vi "Sepios_DepthController_main-for separate Testing.vi"() -> ()   [LabVIEW 2013]
uses:
  <vilib>/myRIO/Instrument Drivers/Utilities/Utilities.lvlib
panel:
  in  "Excessive_Depth_Deviation_Trigger":dbl=0.4
  out "X_Actual [m]":dbl
  out "X_Desired":dbl
  in  "Calibrate Depth":bool
  out "P_ref [Pa]":dbl
  in  "Neutral Buoancy_x":dbl=0.2
  in  "Ti_Depth_Control":dbl=1e-05
  in  "kp_Depth_Control":dbl=0.3
  in  "Integrator enabled range Depth":dbl=0.1
  in  "kp_Motor":dbl=150.0 min=0.0 max=20.0 step=0.01
  in  "Ti_Motor":dbl=1.72e-05 min=0.0 step=0.0001
  in  "Integrator_enable_Range_Motor":dbl=0.03 min=0.0 step=0.01
  out "error out":errorcluster
  in  "STOP":bool
  in  "Tab Control":enum32{"Page 1"}(tab)
  in  "Max Depth":dbl=3.5 max=10.0 step=0.5
  out "Depth [m]":cluster{dbl, dbl, dbl}(slide)={0.0, -0.9890109890109892, 0.0} scale format="%#_3g"
  out "Motor Current[A]":dbl(knob) scale=0.0..3.0
  in  "Depth Desired [m]":dbl min=0.0 step=0.1
  # "Depth Conrol"
  # "SB: Position Control"
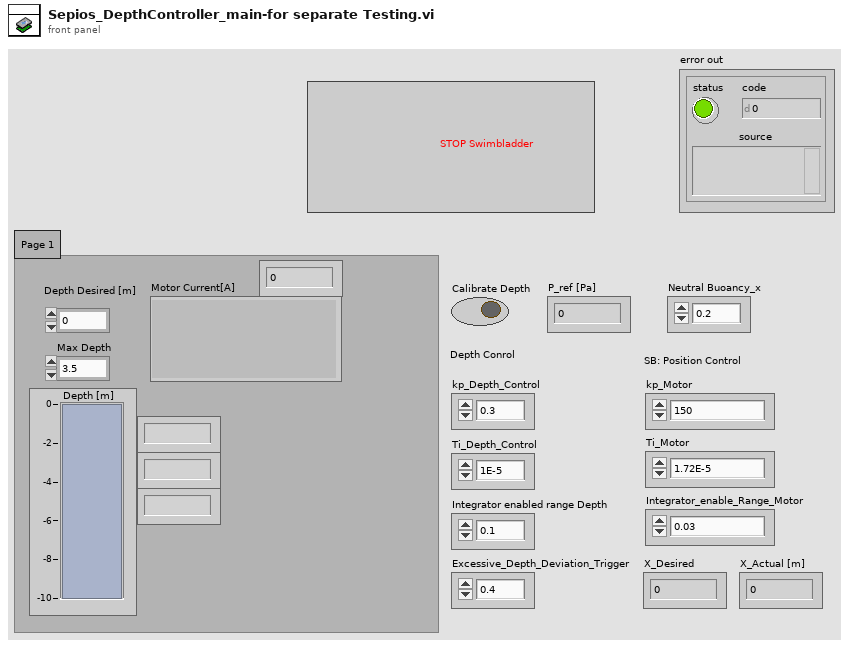
[diagram p1: front panel]
types:
  T1 = cluster{"Water Density":dbl, "SB_parameters":cluster{"x0":dbl, "U_full":dbl, "U_empty":dbl}}
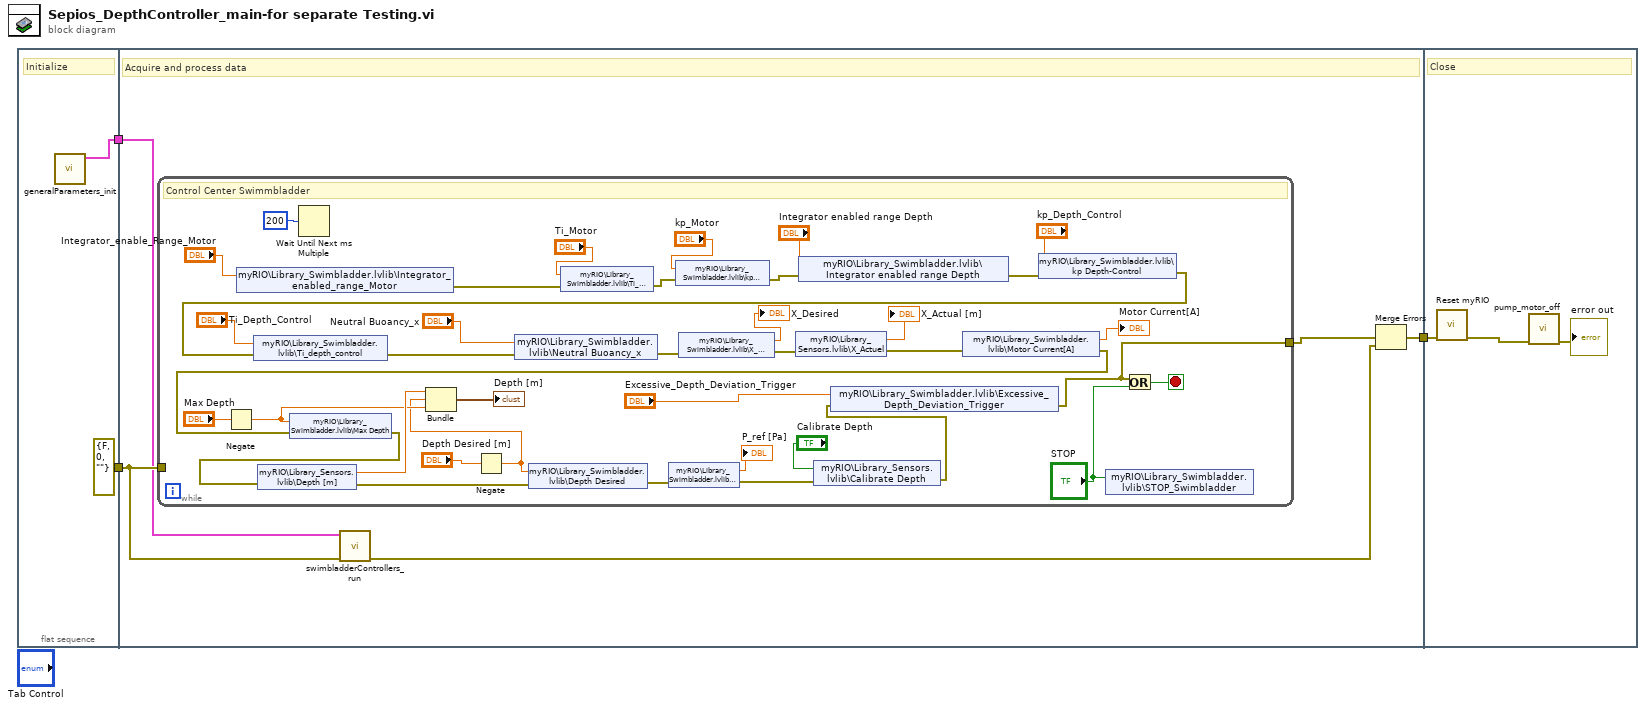
[diagram p0: block diagram]
diagram:
  n1 = flat-sequence {
    tunnel: [errorcluster {"status"=FALSE, "code"=0, "source"=""} ("error out")] -> w3
    tunnel: [w4] -> w2
    tunnel: w3 -> [w8]
    tunnel: w2 -> [w6]
    tunnel: [w10] -> w1
    tunnel: w1 -> [w51]
    frame #0 {
      # "Initialize"
      n2 = call "generalParameters_init.vi"() -> ("General Parameters"=w4:T1)  [unwired: 11 in]
    }
    frame #1 {
      # "Acquire and process data"
      n3 = while {
        tunnel: w8 -> [_]
        tunnel: [w12] -> w7
        stop <- w47 stop-if-true
        # "Control Center Swimmbladder"
        n4 = Negate(x="Max Depth") -> (-x=w15:dbl)
        n5 = shared-variable "myRIO\\Library_Swimbladder.lvlib\\Integrator_enabled_range_Motor"("Integrator_enable_Range_Motor") -> (error out=w41:errorcluster)  [unwired: 1 in]
        n6 = Wait Until Next ms Multiple(millisecond multiple=u32 200) -> ()  [unwired: 1 out]
        n7 = Negate(x="Depth Desired [m]") -> (-x=w14:dbl)
        n8 = shared-variable "myRIO\\Library_Swimbladder.lvlib\\Ti_Motor"("Ti_Motor", error in=w41) -> (error out=w40:errorcluster)
        n9 = shared-variable "myRIO\\Library_Swimbladder.lvlib\\kp Motor"("kp_Motor", error in=w40) -> (error out=w38:errorcluster)
        n10 = shared-variable "myRIO\\Library_Swimbladder.lvlib\\Integrator enabled range Depth"("Integrator enabled range Depth", error in=w38) -> (error out=w37:errorcluster)
        n11 = shared-variable "myRIO\\Library_Swimbladder.lvlib\\kp Depth-Control"("kp_Depth_Control", error in=w37) -> (error out=w35:errorcluster)
        n12 = shared-variable "myRIO\\Library_Swimbladder.lvlib\\Ti_depth_control"("Ti_Depth_Control", error in=w35) -> (error out=w33:errorcluster)
        n13 = shared-variable "myRIO\\Library_Swimbladder.lvlib\\Neutral Buoancy_x"("Neutral Buoancy_x", error in=w33) -> (error out=w31:errorcluster)
        n14 = shared-variable "myRIO\\Library_Swimbladder.lvlib\\X_Desired"(error in=w31) -> (→"X_Desired":dbl, error out=w29:errorcluster)
        n15 = shared-variable "myRIO\\Library_Sensors.lvlib\\X_Actuel"(error in=w29) -> (→"X_Actual [m]":dbl, error out=w28:errorcluster)
        n16 = shared-variable "myRIO\\Library_Swimbladder.lvlib\\Motor Current[A]"(error in=w28) -> (→"Motor Current[A]":dbl, error out=w19:errorcluster)
        n17 = shared-variable "myRIO\\Library_Swimbladder.lvlib\\Max Depth"(w15, error in=w19) -> (error out=w18:errorcluster)
        n18 = shared-variable "myRIO\\Library_Sensors.lvlib\\Depth [m]"(error in=w18) -> (w20:dbl, error out=w26:errorcluster)
        n19 = Bundle("Double"=w20, w14, w15) -> (→"Depth [m]":cluster{"Double":dbl, dbl, dbl})  [unwired: 1 in]
        n20 = shared-variable "myRIO\\Library_Swimbladder.lvlib\\Depth Desired"(w14, error in=w26) -> (error out=w24:errorcluster)
        n21 = shared-variable "myRIO\\Library_Swimbladder.lvlib\\P_ref"(error in=w24) -> (→"P_ref [Pa]":dbl, error out=w23:errorcluster)
        n22 = shared-variable "myRIO\\Library_Sensors.lvlib\\Calibrate Depth"("Calibrate Depth", error in=w23) -> (error out=w13:errorcluster)
        n23 = shared-variable "myRIO\\Library_Swimbladder.lvlib\\Excessive_Depth_Deviation_Trigger"("Excessive_Depth_Deviation_Trigger", error in=w13) -> (error out=w12:errorcluster)
        n24 = shared-variable "myRIO\\Library_Swimbladder.lvlib\\STOP_Swimbladder"("STOP") -> ()  [unwired: 1 in, 1 out]
        n25 = Or(x=w12, y="STOP") -> (x .or. y?=w47:bool)
      }
      n26 = call "swimbladderControllers_run.vi"("error in (no error)"=w8, "General Parameters"=w6) -> ("error out"=w9:errorcluster)  [unwired: 9 in]
      n27 = Merge Errors(w7, w9) -> (w10:errorcluster)  [unwired: 1 in]
    }
    frame #2 {
      # "Close"
      n28 = call <vilib>:"Reset myRIO.vi"("error in (no error)"=w51) -> ("error out"=w50:errorcluster)  [unwired: 10 in]
      n29 = call "pump_motor_off.vi"("error in (no error)"=w50) -> ("error out"=→"error out":errorcluster)  [unwired: 10 in]
    }
  }
